vi "DataVIS_Read WIRING.donkey Data.vi"(8 "error in (no error)":errorcluster, 11 "file path (use dialog)":path) -> (0 "error out":errorcluster, 3 "Wiring Info":string[][](array[string]))   [LabVIEW 2016]
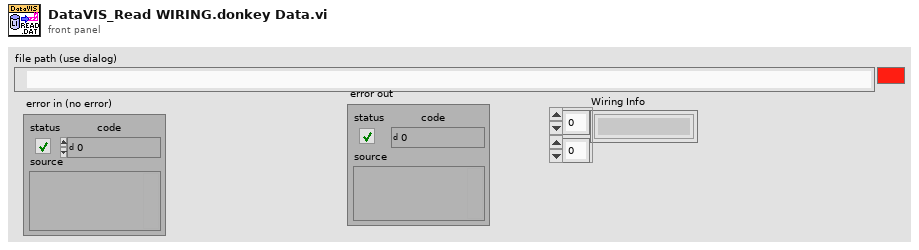
[diagram p1: front panel]
types:
  T1 = enum16{"open", "replace", "create", "open or create", "replace or create", "replace or create with confirmation"}
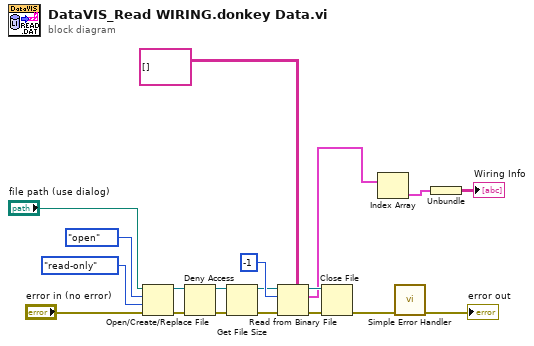
[diagram p0: block diagram]
diagram:
  n1 = Open/Create/Replace File(file path (use dialog)="file path (use dialog)", error in="error in (no error)", operation (0:open)=T1."open", access (0:read/write)=enum16{"read/write", "read-only", "write-only"}."read-only") -> (refnum out=w14:refnum<file>, error out=w13:errorcluster)  [unwired: 2 in, 1 out]
  n2 = Deny Access(4:w13, 7:w14) -> (0:w15:errorcluster, 3:w16:refnum<file>)  [unwired: 1 in]
  n3 = Get File Size(file=w16, error in=w15) -> (refnum out=w7:refnum<file>, 0:w11:errorcluster)  [unwired: 1 out]
  n4 = Read from Binary File(5:string[][] [], 8:w11, 10:-1 ("count (1)"), 11:w7) -> (0:w9:errorcluster, 2:w3:cluster{string[][]}[], 3:w8:refnum<file>)  [unwired: 2 in, 1 out]
  n5 = Close File(refnum=w8, error in=w9) -> (error out=w10:errorcluster)  [unwired: 1 out]
  n6 = Index Array(array=w3) -> (element=w2:cluster{string[][]})  [unwired: 1 in]
  n7 = call <vilib>:"Simple Error Handler.vi"("error in (no error)"=w10) -> ("error out"=→"error out":errorcluster)  [unwired: 4 in, 4 out]
  n8 = Unbundle(w2) -> (→"Wiring Info":string[][])
